vi "FTW-Socket-Construct.vi"(5 "Socket Topology":T1, 7 "Raw Socket?":bool, 9 "Linger":i32=1000 format="%d msec", 11 "error in":errorcluster, 12 "Send Buffer Limit":i32=1024 format="%dkB", 13 "Receive Buffer Limit":i32=1024 format="%dkB") -> (4 "FTW Socket":refnum<class "FTW-Socket.lvclass">, 15 "error out":errorcluster)   [LabVIEW 2013, in "FTW-Socket.lvclass"]
uses:
  FTW-Socket.lvclass
  FTW-Socket-Type.ctl
  FTW-Socket.lvclass/FTW-Socket.ctl
panel:
  # "Inputs"
  # "Outputs"
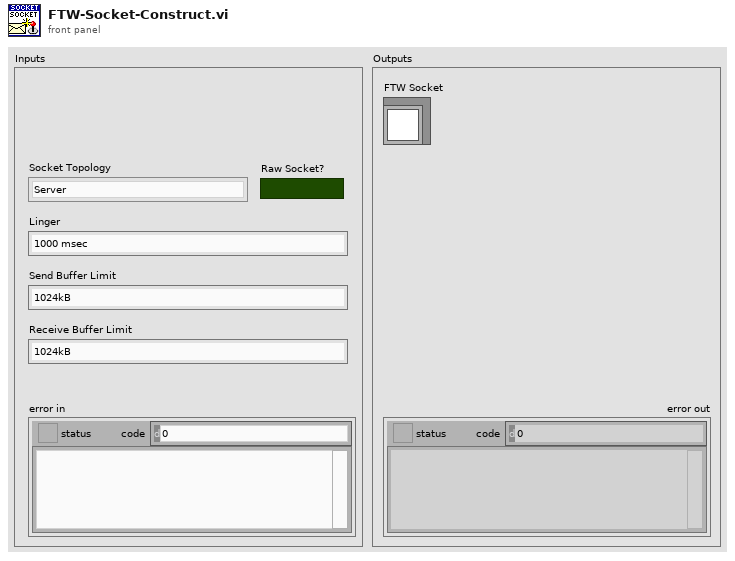
[diagram p1: front panel]
types:
  T1 = typedef "FTW-Socket.lvclass/FTW-Socket-Type.ctl" = enum32{"Server", "Client", "Publisher", "Subscriber", "Pipeline Producer", "Pipeline Consumer", "Surveyor", "Respondent", "Exclusive Pair", "Bus"}
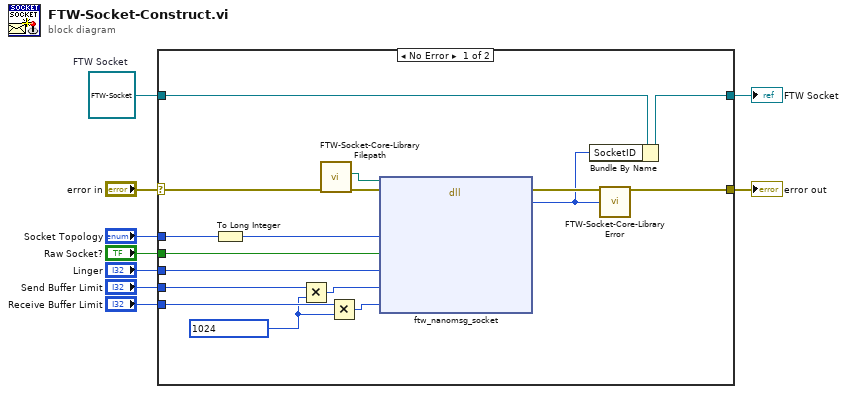
[diagram p0: block diagram]
diagram:
  w5 = refnum<class "FTW-Socket.lvclass"> refnum  # FTW Socket
  n1 = case shown="No Error" "error in" {
    selector: "error in" -> [w26 w28]
    tunnel: [w21 w27] -> w9
    tunnel: [w20 w28] -> w8
    tunnel: "Socket Topology" -> [w18 _]
    tunnel: w5 -> [w25 w27]
    tunnel: "Receive Buffer Limit" -> [w16 _]
    tunnel: "Send Buffer Limit" -> [w15 _]
    tunnel: "Linger" -> [w17 _]
    tunnel: "Raw Socket?" -> [w10 _]
    frame No Error {
      w12 = 1024 ("Receive Buffer Limit")
      n2 = To Long Integer(number=w18) -> (32bit integer=w11:i32)
      n3 = Multiply(x=w15, y=w12) -> (x*y=w14:i32)
      n4 = call "FTW-Socket-Core-LibraryFilepath.vi"("error in"=w26) -> ("error out"=w19:errorcluster, "Library Filepath"=w24:path)  [unwired: 8 in, 1 out]
      n5 = Multiply(x=w16, y=w12) -> (x*y=w13:i32)
      n6 = dll-call lib="?" fn="ftw_nanomsg_socket"(path in=w24, error in=w19, "Scalability Protocol"=w11, "Raw?"=w10, "Linger (msec)"=w17, "Send Buffer (bytes)"=w14, "Receive Buffer (bytes)"=w13) -> (error out=w23:errorcluster, "SocketID"=w22:i64)  [unwired: 8 in, 1 out]
      n7 = Bundle By Name(cluster=w25, "SocketID"=w22) -> (w21:refnum<class "FTW-Socket.lvclass">)
      n8 = call "FTW-Socket-Core-LibraryError.vi"("error in"=w23, "Return Value"=w22) -> ("error out"=w20:errorcluster)  [unwired: 13 in]
    }
    frame Error {
    }
  }
  "error out" <- w8
  "FTW Socket" <- w9
